vi "Read Offset and Multiplier.vi"(9 "GraphScale in":refnum<class "GraphScale.lvclass">) -> (3 "GraphScale out":refnum<class "GraphScale.lvclass">, 4 "Offset and Multiplier":cluster{"Offset":dbl, "Multiplier":dbl})   [LabVIEW 2014, in "Raspberry Pi Compatible Compiler for LabVIEW.lvlib" / "GraphScale.lvclass"]
uses:
  GraphScale.lvclass
  GraphScale.lvclass/GraphScale.ctl
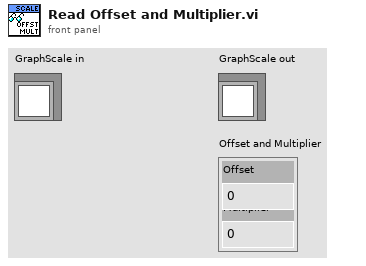
[diagram p1: front panel]
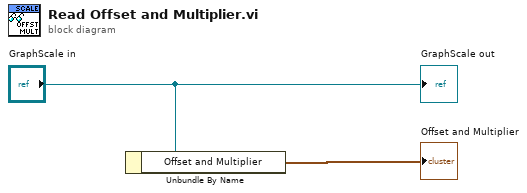
[diagram p0: block diagram]
diagram:
  n1 = Unbundle By Name("GraphScale in") -> ("Offset and Multiplier"=→"Offset and Multiplier":cluster{"Offset":dbl, "Multiplier":dbl})
  "GraphScale out" <- "GraphScale in"
